vi "GetEventForceActuatorStateField.vi"(10 "Event Data":string, 11 "Cluster in":refnum<vi>) -> (3 "Array":string[](array[string]))   [LabVIEW 2016]
uses:
  SALLV_m1m3/DataTypes/logevent_ForceActuatorState.ctl
  SALLV_m1m3/SALLV_m1m3.lvlib
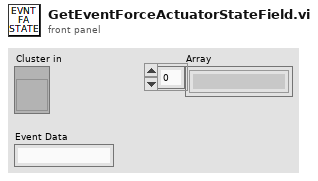
[diagram p1: front panel]
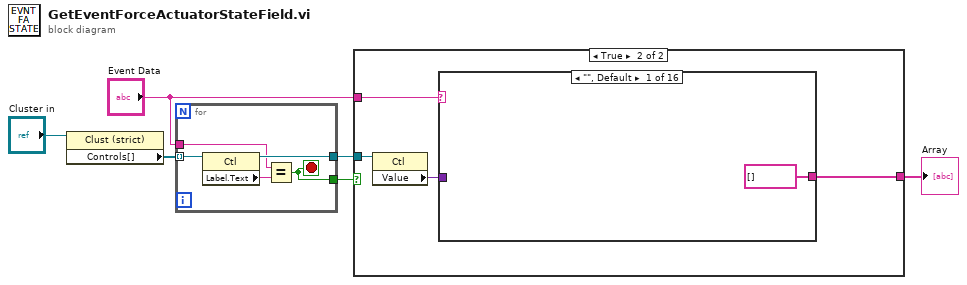
[diagram p0: block diagram]
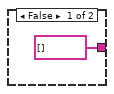
[diagram p2: hidden frame]
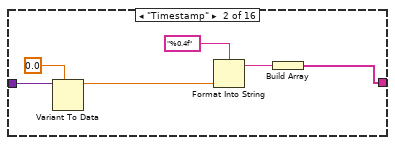
[diagram p3: hidden frame]
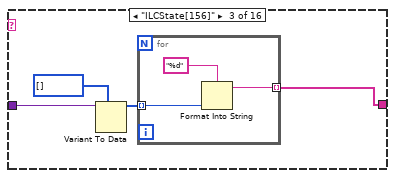
[diagram p4: hidden frame]
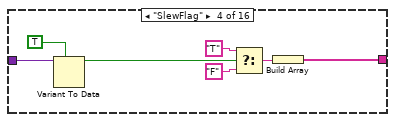
[diagram p5: hidden frame]
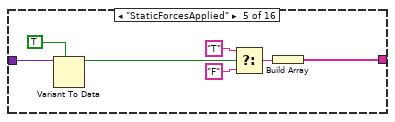
[diagram p6: hidden frame]
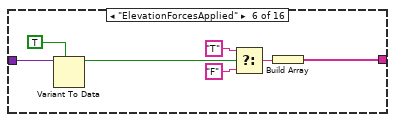
[diagram p7: hidden frame]
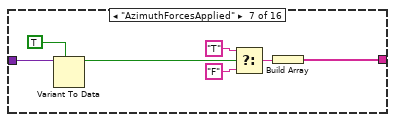
[diagram p8: hidden frame]
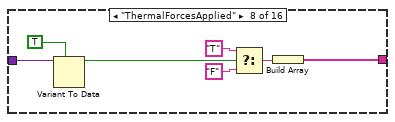
[diagram p9: hidden frame]
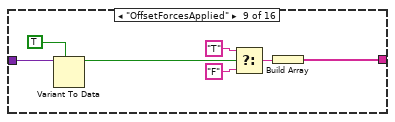
[diagram p10: hidden frame]
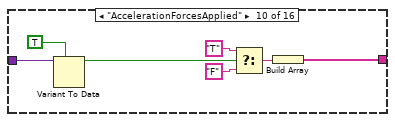
[diagram p11: hidden frame]
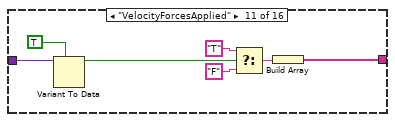
[diagram p12: hidden frame]
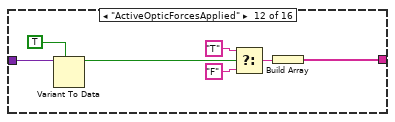
[diagram p13: hidden frame]
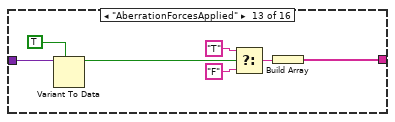
[diagram p14: hidden frame]
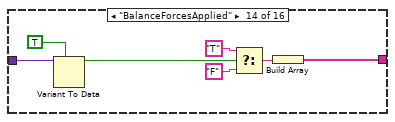
[diagram p15: hidden frame]
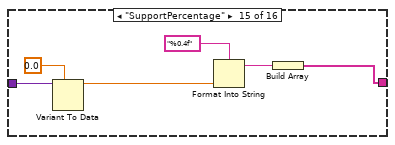
[diagram p16: hidden frame]
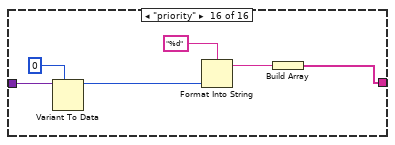
[diagram p17: hidden frame]
diagram:
  n1 = property on="Property Node" class="Clust (strict)"(reference="Cluster in") -> ("Controls[]"=w3:refnum<vi>[])  [unwired: 1 in, 2 out]
  n2 = for {
    tunnel: w3 -> [w11] mode=indexing
    tunnel: [w10] -> w5
    tunnel: "Event Data" -> [w8]
    tunnel: [w7] -> w6
    stop <- w7 stop-if-true
    n3 = property on="Property Node" class="Ctl"(reference=w11) -> (reference out=w10:refnum<vi>, "Label.Text"=w9:string)  [unwired: 1 in, 1 out]
    n4 = Equal?(x=w8, y=w9) -> (x = y?=w7:bool)
  }
  n5 = case shown="True" w6 {
    tunnel: "Event Data" -> [_ w16]
    tunnel: w5 -> [_ w15]
    tunnel: [string[] [] w13] -> w2
    frame False {
    }
    frame True {
      n6 = property on="Property Node" class="Ctl"(reference=w15) -> ("Value"=w14:variant)  [unwired: 1 in, 2 out]
      n7 = case shown="\"\", Default" w16 {
        tunnel: [string[] [] w21 w24 w37 w44 w51 w58 w65 w72 w79 w86 w93 w100 w107 w111 w117] -> w13
        tunnel: w14 -> [_ w19 w27 w36 w43 w50 w57 w64 w71 w78 w85 w92 w99 w106 w109 w115]
        frame "", Default {
        }
        frame "Timestamp" {
          n8 = Variant To Data(type=0.0, Variant=w19) -> (data=w20:dbl)  [unwired: 1 in, 1 out]
          n9 = Format Into String(format string="%0.4f", w20) -> (resulting string=w22:string)  [unwired: 2 in, 1 out]
          n10 = Build Array(w22) -> (w21:string[])
        }
        frame "ILCState[156]" {
          n11 = Variant To Data(type=i16[] [], Variant=w27) -> (data=w25:i16[])  [unwired: 1 in, 1 out]
          n12 = for {
            tunnel: w25 -> [w29] mode=indexing
            tunnel: [w28] -> w24 mode=indexing
            n13 = Format Into String(format string="%d", w29) -> (resulting string=w28:string)  [unwired: 2 in, 1 out]
          }
        }
        frame "SlewFlag" {
          n14 = Variant To Data(type=TRUE, Variant=w36) -> (data=w33:bool)  [unwired: 1 in, 1 out]
          n15 = Select(t="T", s=w33, f="F") -> (s? t:f=w32:string)
          n16 = Build Array(w32) -> (w37:string[])
        }
        frame "StaticForcesApplied" {
          n17 = Variant To Data(type=TRUE, Variant=w43) -> (data=w40:bool)  [unwired: 1 in, 1 out]
          n18 = Select(t="T", s=w40, f="F") -> (s? t:f=w39:string)
          n19 = Build Array(w39) -> (w44:string[])
        }
        frame "ElevationForcesApplied" {
          n20 = Variant To Data(type=TRUE, Variant=w50) -> (data=w47:bool)  [unwired: 1 in, 1 out]
          n21 = Select(t="T", s=w47, f="F") -> (s? t:f=w46:string)
          n22 = Build Array(w46) -> (w51:string[])
        }
        frame "AzimuthForcesApplied" {
          n23 = Variant To Data(type=TRUE, Variant=w57) -> (data=w54:bool)  [unwired: 1 in, 1 out]
          n24 = Select(t="T", s=w54, f="F") -> (s? t:f=w53:string)
          n25 = Build Array(w53) -> (w58:string[])
        }
        frame "ThermalForcesApplied" {
          n26 = Variant To Data(type=TRUE, Variant=w64) -> (data=w61:bool)  [unwired: 1 in, 1 out]
          n27 = Select(t="T", s=w61, f="F") -> (s? t:f=w60:string)
          n28 = Build Array(w60) -> (w65:string[])
        }
        frame "OffsetForcesApplied" {
          n29 = Variant To Data(type=TRUE, Variant=w71) -> (data=w68:bool)  [unwired: 1 in, 1 out]
          n30 = Select(t="T", s=w68, f="F") -> (s? t:f=w67:string)
          n31 = Build Array(w67) -> (w72:string[])
        }
        frame "AccelerationForcesApplied" {
          n32 = Variant To Data(type=TRUE, Variant=w78) -> (data=w75:bool)  [unwired: 1 in, 1 out]
          n33 = Select(t="T", s=w75, f="F") -> (s? t:f=w74:string)
          n34 = Build Array(w74) -> (w79:string[])
        }
        frame "VelocityForcesApplied" {
          n35 = Variant To Data(type=TRUE, Variant=w85) -> (data=w82:bool)  [unwired: 1 in, 1 out]
          n36 = Select(t="T", s=w82, f="F") -> (s? t:f=w81:string)
          n37 = Build Array(w81) -> (w86:string[])
        }
        frame "ActiveOpticForcesApplied" {
          n38 = Variant To Data(type=TRUE, Variant=w92) -> (data=w89:bool)  [unwired: 1 in, 1 out]
          n39 = Select(t="T", s=w89, f="F") -> (s? t:f=w88:string)
          n40 = Build Array(w88) -> (w93:string[])
        }
        frame "AberrationForcesApplied" {
          n41 = Variant To Data(type=TRUE, Variant=w99) -> (data=w96:bool)  [unwired: 1 in, 1 out]
          n42 = Select(t="T", s=w96, f="F") -> (s? t:f=w95:string)
          n43 = Build Array(w95) -> (w100:string[])
        }
        frame "BalanceForcesApplied" {
          n44 = Variant To Data(type=TRUE, Variant=w106) -> (data=w103:bool)  [unwired: 1 in, 1 out]
          n45 = Select(t="T", s=w103, f="F") -> (s? t:f=w102:string)
          n46 = Build Array(w102) -> (w107:string[])
        }
        frame "SupportPercentage" {
          n47 = Variant To Data(type=sgl 0.0, Variant=w109) -> (data=w110:sgl)  [unwired: 1 in, 1 out]
          n48 = Format Into String(format string="%0.4f", w110) -> (resulting string=w112:string)  [unwired: 2 in, 1 out]
          n49 = Build Array(w112) -> (w111:string[])
        }
        frame "priority" {
          n50 = Variant To Data(type=0, Variant=w115) -> (data=w116:i32)  [unwired: 1 in, 1 out]
          n51 = Format Into String(format string="%d", w116) -> (resulting string=w118:string)  [unwired: 2 in, 1 out]
          n52 = Build Array(w118) -> (w117:string[])
        }
      }
    }
  }
  "Array" <- w2
